vi "Motor_generatemotion.vi"(1 "Conversion\n (steps/mm)":dbl[](array[numeric])=[12500.0, 31496.063, 31496.063, 31496.063] format="%#_13g", 2 "Distance  (mm)":dbl[](array[numeric])=[0.0, 0.0, 0.0, 0.0] format="%#_13g") -> (0 "Movement String":string)   [LabVIEW 2018]
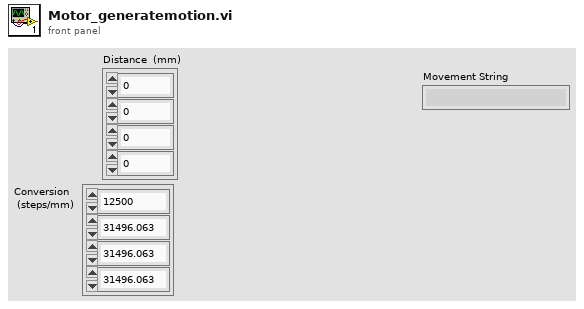
[diagram p1: front panel]
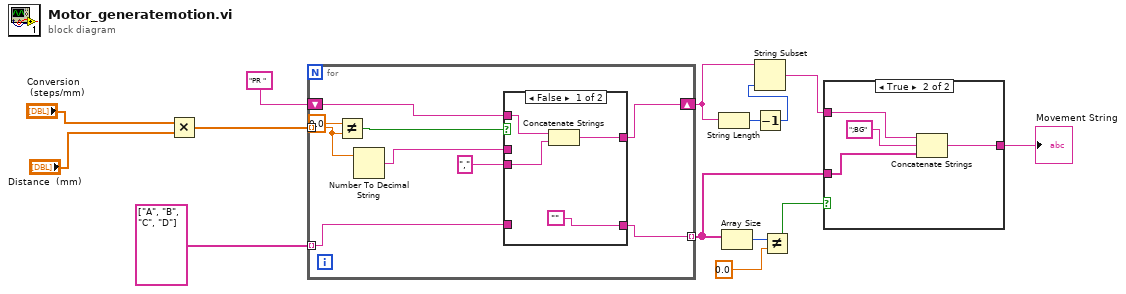
[diagram p0: block diagram]
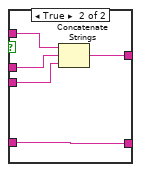
[diagram p3: hidden frame]
diagram:
  n1 = Multiply(x="Conversion\n (steps/mm)", y="Distance  (mm)") -> (x*y=w12:dbl[])
  n2 = for {
    tunnel: w12 -> [w17] mode=indexing
    tunnel: string[] ["A", "B", "C", "D"] -> [w23] mode=indexing
    tunnel: [w20] -> w7 mode=indexing
    shift-right: [w19] -> w4
    shift-left: "PR " ("string") -> [w18]
    n3 = Not Equal?(x=0.0, y=w17) -> (x != y?=w16:bool)
    n4 = Number To Decimal String(number=w17) -> (decimal integer string=w22:string)  [unwired: 1 in]
    n5 = case shown="False" w16 {
      tunnel: w23 -> [_ w32]
      tunnel: ["" w32] -> w20
      tunnel: w22 -> [_ w31]
      tunnel: [w25 w30] -> w19
      tunnel: "," -> [w24 w29]
      tunnel: w18 -> [w26 w28]
      frame False {
        n6 = Concatenate Strings(w26, w24) -> (w25:string)
      }
      frame True {
        n7 = Concatenate Strings(w28, w31, w29) -> (w30:string)
      }
    }
  }
  n8 = String Length(string=w4) -> (length=w3:i32)
  n9 = Array Size(array=w7) -> (size(s)=w9:i32)
  n10 = Decrement(x=w3) -> (x-1=w2:i32)
  n11 = String Subset(string=w4, length (rest)=w2) -> (substring=w1:string)  [unwired: 1 in]
  n12 = Not Equal?(x=w9, y=0.0) -> (x != y?=w10:bool)
  n13 = case shown="True" w10 {
    tunnel: w7 -> [_ w36]
    tunnel: w1 -> [w33 w37]
    tunnel: [w33 w34] -> w6
    frame False {
    }
    frame True {
      n14 = Concatenate Strings(w37, ";BG" ("string"), w36) -> (w34:string)
    }
  }
  "Movement String" <- w6
